vi "MULTI_csv.vi"() -> ()   [LabVIEW 2017]
uses:
  <vilib>/Utility/file.llb/Write Delimited Spreadsheet (string).vi
panel:
  in  "COMPILADO":path
  in  "HEAD":string[](array[string])=["inicios", "finales", "etiquetas"]
  in  "Boolean 6":bool
  in  "Path 6":path
  in  "?":enum32{"PREVIAS", "TOTAL"}(tab)
  out "Lectura CSV - clase 6":string[][](array[string])
  out "Lectura CSV - clase 1":string[][](array[string])
  out "Lectura CSV - clase 2":string[][](array[string])
  out "Lectura CSV - clase 3":string[][](array[string])
  out "Lectura CSV - clase 4":string[][](array[string])
  out "Lectura CSV - clase 5":string[][](array[string])
  out "Array":string[][](array[string])
  in  "Boolean 5":bool
  in  "Boolean  4":bool
  in  "Boolean 3":bool
  in  "Boolean 2":bool
  in  "Boolean 1":bool=TRUE
  in  "Path 5":path
  in  "Path 4":path
  in  "Path 3":path
  in  "Path 2":path
  in  "Path":path
  # "Primero Cargue los archivos de entrada, verifíquelos y luego corra en TOTAL"
  # "SELECTOR DE ZONAS CLASIFICADAS"
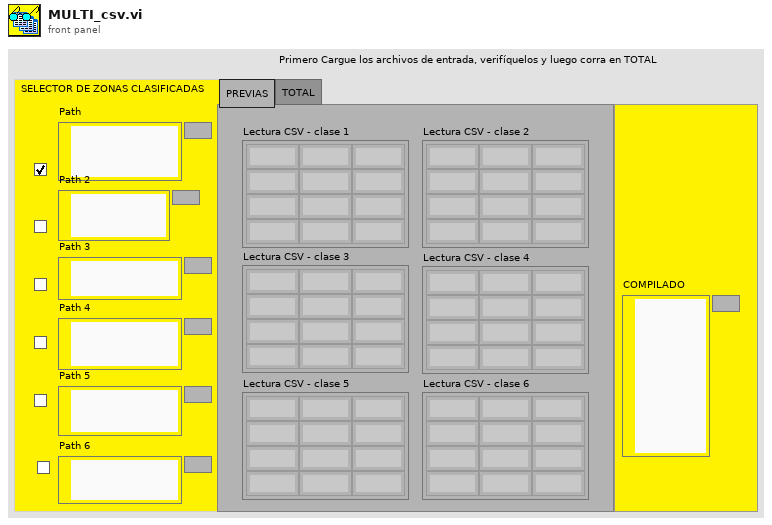
[diagram p1: front panel]
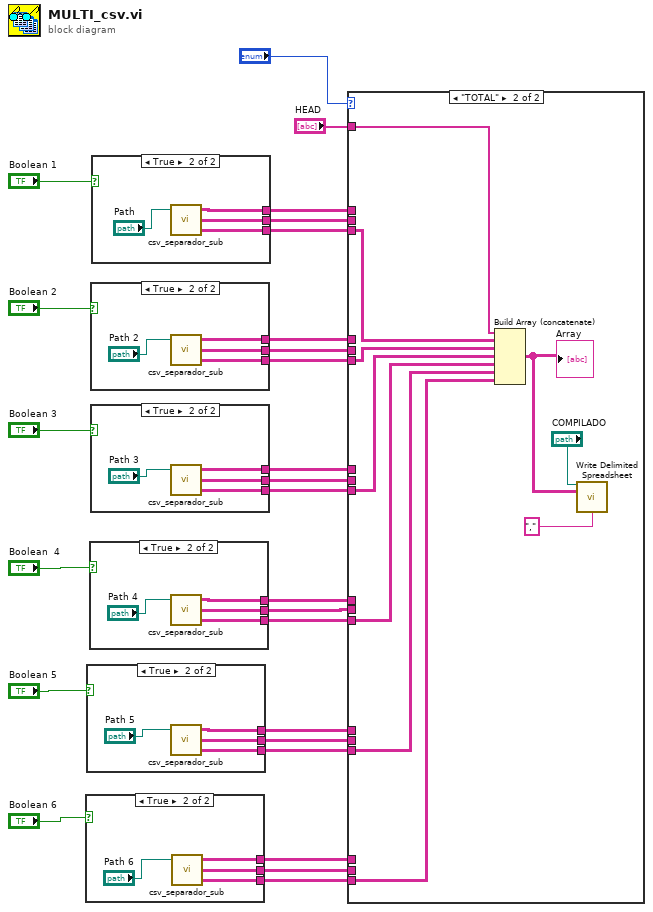
[diagram p0: block diagram]
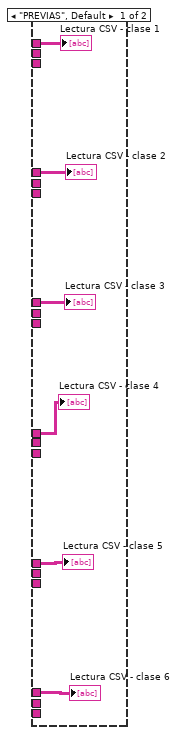
[diagram p2: hidden frame]
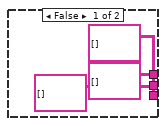
[diagram p3: hidden frame]
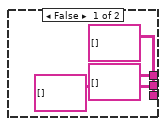
[diagram p4: hidden frame]
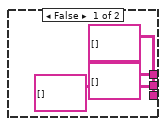
[diagram p5: hidden frame]
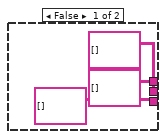
[diagram p6: hidden frame]
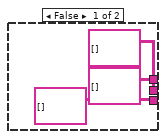
[diagram p7: hidden frame]
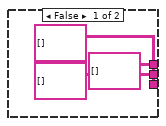
[diagram p8: hidden frame]
diagram:
  n1 = case shown="True" "Boolean 6" {
    tunnel: [string[][] [] ("all rows") w32] -> w14
    tunnel: [string[][] [] ("subarray 2") w31] -> w3
    tunnel: [string[][] [] ("subarray") w30] -> w2
    frame False {
    }
    frame True {
      n2 = call "csv_separador_sub.vi"("Archivo de referencias (.csv)"="Path 6") -> ("subarray 2"=w30:string[][], "subarray"=w31:string[][], "all rows"=w32:string[][])  [unwired: 2 in]
    }
  }
  n3 = case shown="True" "Boolean 5" {
    tunnel: [string[][] [] ("all rows") w39] -> w15
    tunnel: [string[][] [] ("subarray 2") w38] -> w5
    tunnel: [string[][] [] ("subarray") w37] -> w4
    frame False {
    }
    frame True {
      n4 = call "csv_separador_sub.vi"("Archivo de referencias (.csv)"="Path 5") -> ("subarray 2"=w37:string[][], "subarray"=w38:string[][], "all rows"=w39:string[][])  [unwired: 2 in]
    }
  }
  n5 = case shown="True" "Boolean  4" {
    tunnel: [string[][] [] ("all rows") w46] -> w16
    tunnel: [string[][] [] ("subarray 2") w45] -> w7
    tunnel: [string[][] [] ("subarray") w44] -> w6
    frame False {
    }
    frame True {
      n6 = call "csv_separador_sub.vi"("Archivo de referencias (.csv)"="Path 4") -> ("subarray 2"=w44:string[][], "subarray"=w45:string[][], "all rows"=w46:string[][])  [unwired: 2 in]
    }
  }
  n7 = case shown="True" "Boolean 2" {
    tunnel: [string[][] [] ("all rows") w53] -> w18
    tunnel: [string[][] [] ("subarray 2") w52] -> w11
    tunnel: [string[][] [] ("subarray") w51] -> w10
    frame False {
    }
    frame True {
      n8 = call "csv_separador_sub.vi"("Archivo de referencias (.csv)"="Path 2") -> ("subarray 2"=w51:string[][], "subarray"=w52:string[][], "all rows"=w53:string[][])  [unwired: 2 in]
    }
  }
  n9 = case shown="True" "Boolean 3" {
    tunnel: [string[][] [] ("all rows") w60] -> w17
    tunnel: [string[][] [] ("subarray 2") w59] -> w9
    tunnel: [string[][] [] ("subarray") w58] -> w8
    frame False {
    }
    frame True {
      n10 = call "csv_separador_sub.vi"("Archivo de referencias (.csv)"="Path 3") -> ("subarray 2"=w58:string[][], "subarray"=w59:string[][], "all rows"=w60:string[][])  [unwired: 2 in]
    }
  }
  n11 = case shown="True" "Boolean 1" {
    tunnel: [string[][] [] ("all rows") w67] -> w19
    tunnel: [string[][] [] ("subarray 2") w66] -> w13
    tunnel: [string[][] [] ("subarray") w65] -> w12
    frame False {
    }
    frame True {
      n12 = call "csv_separador_sub.vi"("Archivo de referencias (.csv)"="Path") -> ("subarray 2"=w65:string[][], "subarray"=w66:string[][], "all rows"=w67:string[][])  [unwired: 2 in]
    }
  }
  n13 = case shown="\"TOTAL\"" "?" {
    tunnel: w19 -> [w74 _]
    tunnel: w18 -> [w73 _]
    tunnel: w17 -> [w72 _]
    tunnel: w16 -> [w71 _]
    tunnel: w15 -> [w70 _]
    tunnel: w14 -> [w69 _]
    tunnel: w13 -> [_ _]
    tunnel: w12 -> [_ w84]
    tunnel: w11 -> [_ _]
    tunnel: w10 -> [_ w83]
    tunnel: w9 -> [_ _]
    tunnel: w8 -> [_ w82]
    tunnel: w7 -> [_ _]
    tunnel: w6 -> [_ w77]
    tunnel: w5 -> [_ _]
    tunnel: w4 -> [_ w76]
    tunnel: w3 -> [_ _]
    tunnel: w2 -> [_ w81]
    tunnel: "HEAD" -> [_ w80]
    frame "PREVIAS", Default {
      "Lectura CSV - clase 6" <- w69
      "Lectura CSV - clase 5" <- w70
      "Lectura CSV - clase 4" <- w71
      "Lectura CSV - clase 3" <- w72
      "Lectura CSV - clase 2" <- w73
      "Lectura CSV - clase 1" <- w74
    }
    frame "TOTAL" {
      n14 = Build Array (concatenate)(w80, w84, w83, w82, w77, w76, w81) -> (w75:string[][])
      "Array" <- w75
      n15 = call-poly <vilib>:"Write Delimited Spreadsheet.vi"("file path (dialog if empty)"="COMPILADO", "2D data"=w75, "delimiter (\\t)"="," ("delimiter (\\t)")) -> ()  [unwired: 11 in, 2 out]
    }
  }
